vi "Read Power Meter.lvclass.vi"(11 "Harmonics in":refnum<class "Harmonics.lvclass">) -> (2 "Power Meter classes":refnum<class "Power Meter.lvclass">[](array[class]), 3 "Harmonics out":refnum<class "Harmonics.lvclass">)   [LabVIEW 2020, in "Harmonics.lvclass"]
uses:
  Harmonics.lvclass
  Instruments/Power Meter/Power Meter.lvclass
  Harmonics.lvclass/Harmonics.ctl
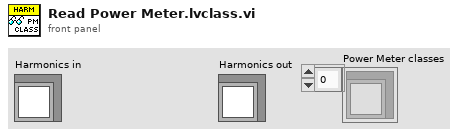
[diagram p1: front panel]
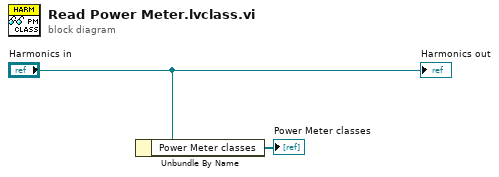
[diagram p0: block diagram]
diagram:
  n1 = Unbundle By Name("Harmonics in") -> ("Power Meter classes"=→"Power Meter classes":refnum<class "Power Meter.lvclass">[])
  "Harmonics out" <- "Harmonics in"
